vi "temp.vi"() -> ()   [LabVIEW 2018]
uses:
  <vilib>/Analysis/Matrix/Datatypes/RealMatrix.ctl
  <vilib>/myRIO/Common/Instrument Driver Framework/myRIO v1.0/PWM/vis/myRIO v1.1 Open PWM.vi
  <vilib>/myRIO/Common/Instrument Driver Framework/myRIO v1.0/PWM/vis/myRIO v1.2 Open PWM.vi
  <vilib>/myRIO/Common/Instrument Driver Framework/roboRIO v1.0/PWM/vis/roboRIO v1.0 Open PWM.vi
  <vilib>/myRIO/Common/Instrument Driver Framework/EL-RIO-CM v1.0/PWM/vis/EL-RIO-CM v1.0 Open PWM.vi
  <vilib>/myRIO/Common/Instrument Driver Framework/ELVIS III v1.0/PWM/vis/ELVIS III v1.1 Open PWM.vi
  <vilib>/myRIO/Common/Instrument Driver Framework/myRIO v1.0/UART/vis/myRIO v1.0 Close UART.vi
  <vilib>/myRIO/Common/Instrument Driver Framework/Utilities/vis/Validate Channels.vi
  <vilib>/myRIO/Common/Instrument Driver Framework/myRIO v1.0/PWM/vis/myRIO v1.0 Reserve PWM.vi
  <vilib>/myRIO/Common/Instrument Driver Framework/roboRIO v1.0/PWM/vis/roboRIO v1.0 Reserve PWM.vi
  <vilib>/myRIO/Common/Instrument Driver Framework/ELVIS III v1.0/PWM/vis/ELVIS III v1.0 Reserve PWM.vi
  <vilib>/myRIO/Common/Instrument Driver Framework/myRIO v1.0/PWM/vis/myRIO v1.0 Build MUX Configuration PWM.vi
  <vilib>/myRIO/Common/Instrument Driver Framework/myRIO v1.0/Resource Manager/vis/myRIO v1.0 Reserve Channel List.vi
  <vilib>/myRIO/Common/Instrument Driver Framework/roboRIO v1.0/PWM/vis/roboRIO v1.0 Build MUX Configuration PWM.vi
  <vilib>/myRIO/Common/Instrument Driver Framework/roboRIO v1.0/Resource Manager/vis/roboRIO v1.0 Reserve Channel List.vi
  <vilib>/myRIO/Common/Instrument Driver Framework/ELVIS III v1.0/Resource Manager/vis/ELVIS III v1.0 Reserve Channel List.vi
  <vilib>/myRIO/Common/Instrument Driver Framework/ELVIS III v1.0/PWM/vis/ELVIS III v1.0 Build MUX Configuration PWM.vi
  <vilib>/myRIO/Common/Instrument Driver Framework/myRIO v1.0/Resource Manager/vis/myRIO v1.0 Create Configuration List.vi
  <vilib>/myRIO/Common/Instrument Driver Framework/myRIO v1.0/Resource Manager/vis/myRIO v1.0 Reserve Channel.vi
  <vilib>/myRIO/Common/Instrument Driver Framework/myRIO v1.0/Resource Manager/vis/myRIO v1.0 Unreserve Channel.vi
  <vilib>/myRIO/Common/Instrument Driver Framework/roboRIO v1.0/Resource Manager/vis/roboRIO v1.0 Create Configuration List.vi
  <vilib>/myRIO/Common/Instrument Driver Framework/roboRIO v1.0/Resource Manager/vis/roboRIO v1.0 Reserve Channel.vi
  <vilib>/myRIO/Common/Instrument Driver Framework/roboRIO v1.0/Resource Manager/vis/roboRIO v1.0 Unreserve Channel.vi
  <vilib>/myRIO/Common/Instrument Driver Framework/ELVIS III v1.0/Resource Manager/vis/ELVIS III v1.0 Reserve Channel.vi
  <vilib>/myRIO/Common/Instrument Driver Framework/ELVIS III v1.0/Resource Manager/vis/ELVIS III v1.0 Unreserve Channel.vi
  <vilib>/myRIO/Common/Instrument Driver Framework/ELVIS III v1.0/Resource Manager/vis/ELVIS III v1.0 Create Configuration List.vi
  <vilib>/myRIO/Common/Instrument Driver Framework/myRIO v1.0/Resource Manager/vis/myRIO v1.0 Build Mutex Name.vi
  <vilib>/myRIO/Common/Instrument Driver Framework/roboRIO v1.0/Resource Manager/vis/roboRIO v1.0 Build Mutex Name.vi
  <vilib>/myRIO/Common/Instrument Driver Framework/ELVIS III v1.0/Resource Manager/vis/ELVIS III v1.0 Build Mutex Name.vi
  <vilib>/myRIO/Common/Instrument Driver Framework/Utilities/vis/Set_Get Target Info.vi
  <vilib>/Utility/error.llb/Error Cluster From Error Code.vi
  <vilib>/Utility/VariantDataType/GetNumericInfo.vi
  <vilib>/myRIO/Common/Instrument Driver Framework/myRIO v1.0/myRIO v1.1 Open.vi
  <vilib>/myRIO/Common/Instrument Driver Framework/Utilities/vis/IO Manager.vi
  <vilib>/myRIO/Common/Instrument Driver Framework/Utilities/vis/Configuration Manager.vi
  <vilib>/myRIO/Common/Instrument Driver Framework/myRIO v1.0/Resource Manager/vis/myRIO v1.0 Configure IO.vi
  <vilib>/myRIO/Common/Instrument Driver Framework/myRIO v1.0/myRIO v1.0 Close.vi
  <vilib>/myRIO/Common/Instrument Driver Framework/myRIO v1.0/myRIO v1.2 Open.vi
  <vilib>/myRIO/Common/Instrument Driver Framework/roboRIO v1.0/roboRIO v1.0 Open.vi
  <vilib>/myRIO/Common/Instrument Driver Framework/roboRIO v1.0/Resource Manager/vis/roboRIO v1.0 Configure IO.vi
  <vilib>/myRIO/Common/Instrument Driver Framework/EL-RIO-CM v1.0/EL-RIO-CM v1.0 Open.vi
  <vilib>/myRIO/Common/Instrument Driver Framework/ELVIS III v1.0/ELVIS III v1.1 Open.vi
  <vilib>/myRIO/Common/Instrument Driver Framework/ELVIS III v1.0/Resource Manager/vis/ELVIS III v1.0 Configure IO.vi
  <vilib>/myRIO/Common/Instrument Driver Framework/myRIO v1.0/PWM/vis/myRIO v1.0 Write PWM.vi
  <vilib>/myRIO/Common/Instrument Driver Framework/roboRIO v1.0/PWM/vis/roboRIO v1.0 Write PWM.vi
  <vilib>/myRIO/Common/Instrument Driver Framework/ELVIS III v1.0/PWM/vis/ELVIS III v1.0 Write PWM.vi
  <vilib>/myRIO/Common/Instrument Driver Framework/Utilities/vis/FPGA Ref Manager.vi
  <vilib>/myRIO/Common/Instrument Driver Framework/myRIO v1.0/IRQ/vis/myRIO v1.0 IRQ Info FGV.vi
  <vilib>/myRIO/Common/Instrument Driver Framework/myRIO v1.0/IRQ/vis/myRIO v1.0 Timer IRQ Info FGV.vi
  <vilib>/myRIO/Instrument Drivers/Utilities/Utilities.lvlib
  <vilib>/myRIO/Instrument Drivers/Onboard IO/PWM/PWM.lvlib
  <vilib>/Analysis/Matrix/NI_Matrix.lvlib
panel:
  out "offset [%FS] 2":dbl
  in  "null offset 2":bool
  out "duty cycle [%] 2":dbl
  out "pulse width [ms] 2":dbl=1.5
  in  "freq [Hz] 2":dbl=50.0
  in  "[ESC] 2":bool
  out "offset [%FS]":dbl
  in  "null offset":bool
  out "duty cycle [%]":dbl
  out "pulse width [ms]":dbl=1.5
  in  "freq [Hz]":dbl=50.0
  in  "[ESC]":bool
  in  "PWM channel 2":tag="B/PWM0"
  in  "PWM channel":tag="B/PWM0"
  out "arm picture":refnum<vi>(3d-picture)
  out "A x B 3":T1=[[1.0, 0.0, 0.0, 0.0], [0.0, 6.123233995736766e-17, 1.0, 0.0], [0.0, -1.0, 6.123233995736766e-17, 0.0], [0.0, 0.0, 0.0, 1.0]] format="%#_2g"
  out "drawing":refnum<vi>(3d-picture)
  out "x arrya":dbl[][](array[numeric])
  out "phi array":dbl[][](array[numeric])
  out "third array":dbl[][](array[numeric])
  out "second array":dbl[][](array[numeric])
  out "first":dbl[][](array[numeric])
  in  "Enter initials":string
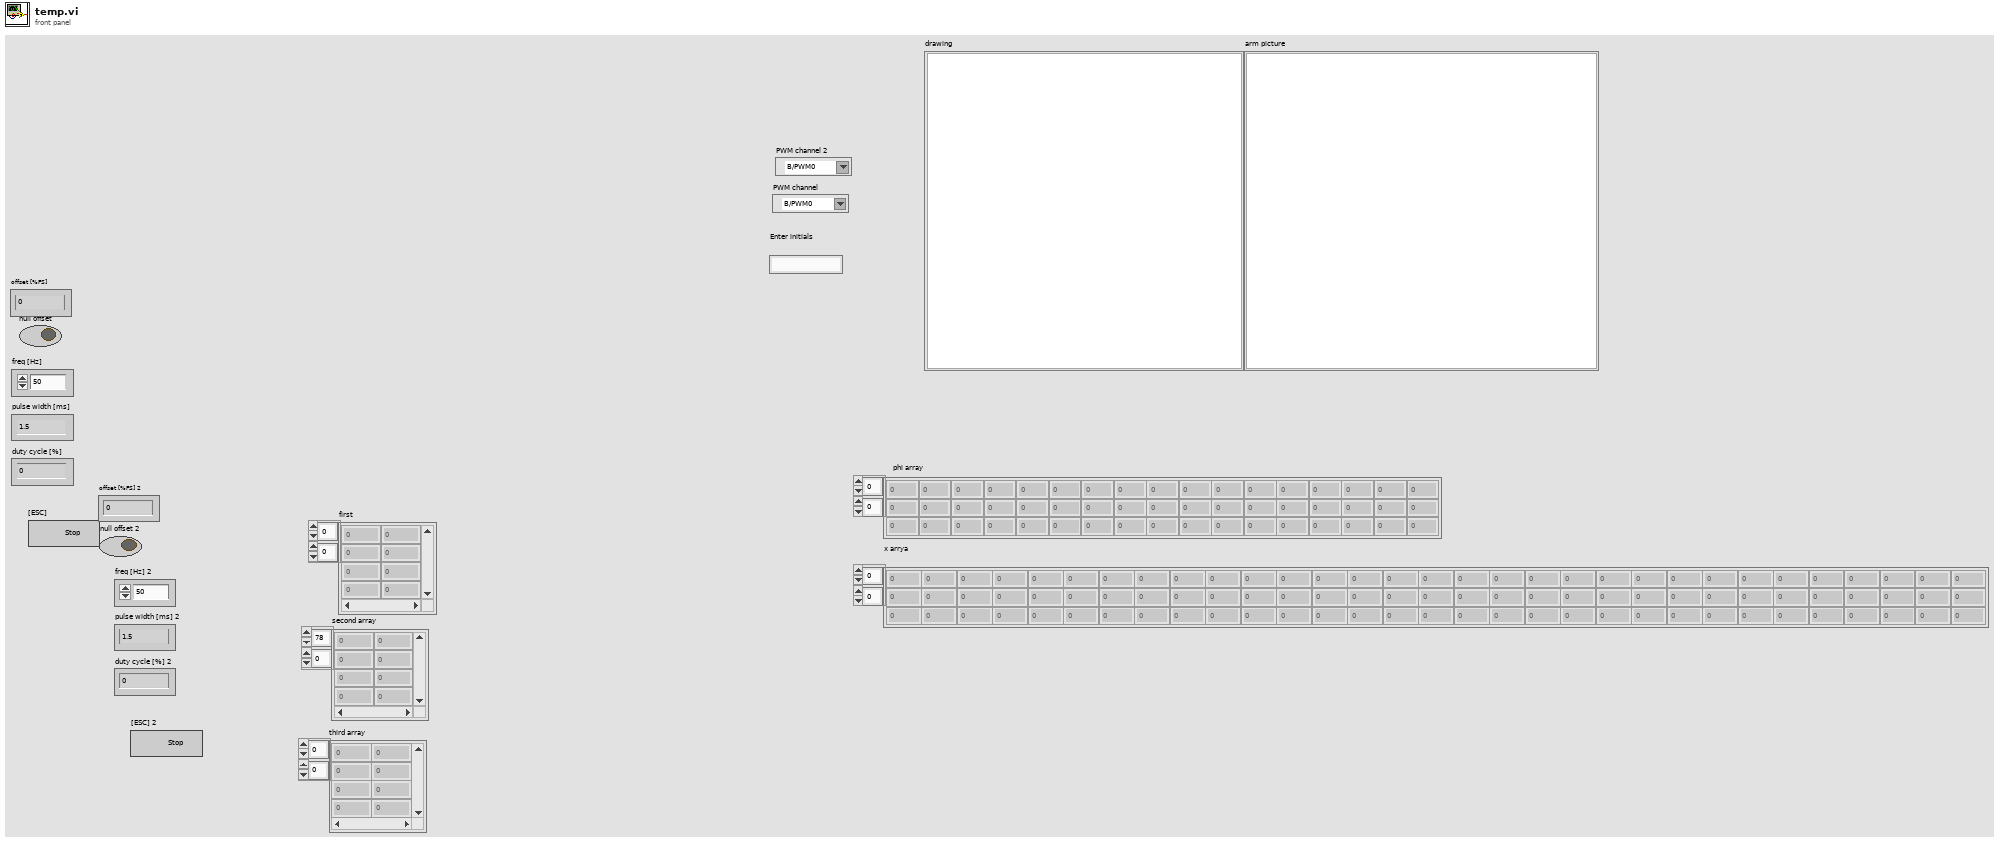
[diagram p1: front panel]
types:
  T1 = typedef "NI_Matrix.lvlib/RealMatrix.ctl" = dbl[][]
  T2 = cluster{"Theta":dbl, "d":dbl, "a":dbl, "alpha (degrees)":dbl}[]
  T3 = cluster{"Theta":dbl, "d":dbl, "a":dbl, "alpha (degrees)":dbl}
  T4 = typedef "PWM.lvlib/PWM Reference.ctl" = cluster{"myRIO Reference":T5, "PWM Channels Enum":T9, "PWM Configuration":T10}
  T5 = typedef "myRIO Generic Hardware Reference.ctl" = cluster{"myRIO Model":T6, "myRIO Hardware Reference":T7}
  T6 = typedef "Hardware Version Enum.ctl" = enum16{"Unknown", "myRIO-1900", "myRIO-1950", "roboRIO", "NI ELVIS RIO CM", "ELVIS III"}
  T7 = typedef "myRIO v1.0 Reference.ctl" = cluster{"Generic FPGA Reference":T8, "Allow multiple opens":bool}
  T8 = typedef "Generic FPGA Reference.ctl" = refnum<k20>
  T9 = typedef "PWM Channels Enum.ctl" = enum16{"Not Connected", "C/PWM0", "C/PWM1", "A/PWM0", "A/PWM1", "A/PWM2", "A/PWM3", "A/PWM4", "A/PWM5", "A/PWM6", "A/PWM7", "A/PWM8", "A/PWM9", "A/PWM10", "A/PWM11", "A/PWM12", "A/PWM13", "A/PWM14", "A/PWM15", "A/PWM16", "A/PWM17", "A/PWM18", "A/PWM19", "B/PWM0", "B/PWM1", "B/PWM2", "B/PWM3", "B/PWM4", "B/PWM5", "B/PWM6", "B/PWM7", "B/PWM8", "B/PWM9", "B/PWM10", "B/PWM11", "B/PWM12", "B/PWM13", "B/PWM14", "B/PWM15", "B/PWM16", "B/PWM17", "B/PWM18", "B/PWM19", "PWM/PWM0", "PWM/PWM1", "PWM/PWM2", "PWM/PWM3", "PWM/PWM4", "PWM/PWM5", "PWM/PWM6", "PWM/PWM7", "PWM/PWM8", "PWM/PWM9"}
  T10 = typedef "PWM.lvlib/PWM Configuration.ctl" = cluster{"Frequency":dbl, "Duty Cycle":dbl}
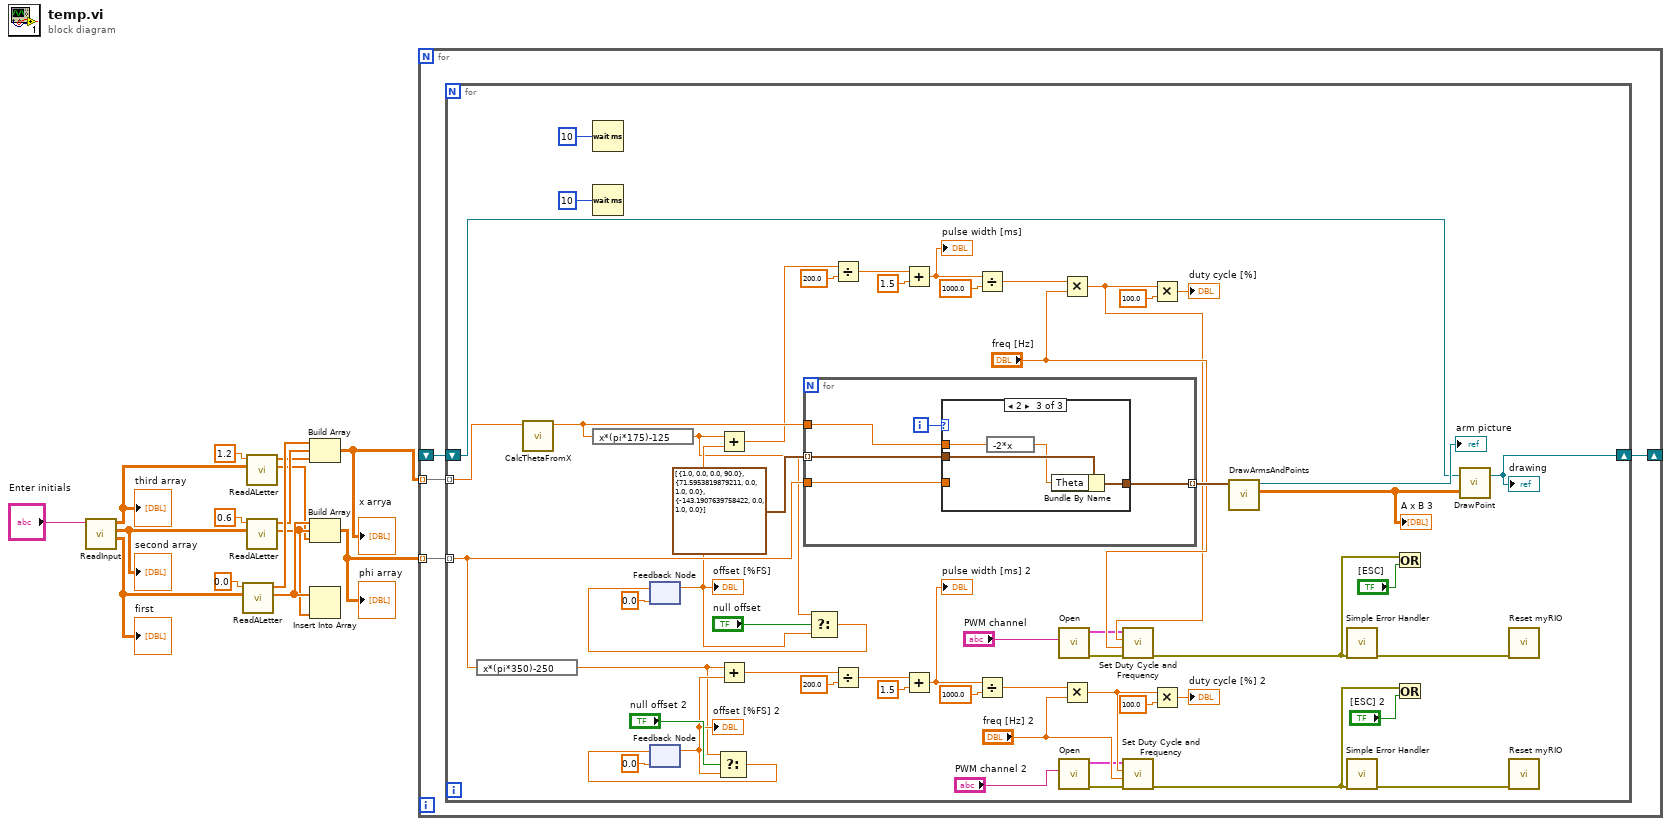
[diagram p0: block diagram]
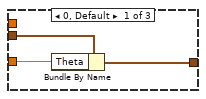
[diagram p2: hidden frame]
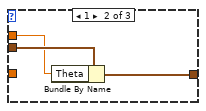
[diagram p3: hidden frame]
diagram:
  n1 = call "ReadInput.vi"("Enter initials"="Enter initials") -> ("all rows 3"=w13:dbl[][], "all rows 2"=w11:dbl[][], "all rows"=w9:dbl[][])  [unwired: 8 in]
  "first" <- w13
  "second array" <- w11
  "third array" <- w9
  n2 = call "ReadALetter.vi"("all rows 3"=w13, "x"=0.0) -> ("Array 3"=w3:dbl[], "Array 4"=w8:dbl[])  [unwired: 8 in]
  n3 = call "ReadALetter.vi"("all rows 3"=w9, "x"=1.2) -> ("Array 3"=w1:dbl[], "Array 4"=w6:dbl[])  [unwired: 8 in]
  n4 = call "ReadALetter.vi"("all rows 3"=w11, "x"=0.6) -> ("Array 3"=w2:dbl[], "Array 4"=w7:dbl[])  [unwired: 8 in]
  n5 = Build Array(w8, w7, w6) -> (w4:dbl[][])
  "x arrya" <- w4
  n6 = Build Array(w3, w2, w1) -> (w5:dbl[][])
  "phi array" <- w5
  n7 = Insert Into Array(array=w3, new element=w2) -> ()  [unwired: 1 in, 1 out]
  n8 = for {
    tunnel: w5 -> [w18] mode=indexing
    shift-right: [w19] -> _
    shift-left: _ -> [w16]
    tunnel: w4 -> [w17] mode=indexing
    n9 = for {
      tunnel: w18 -> [w62] mode=indexing
      tunnel: w17 -> [w69] mode=indexing
      shift-right: [w71] -> w19
      shift-left: w16 -> [w68]
      n10 = expression code="x*(pi*350)-250"(w62) -> (w23:dbl)
      n11 = call "CalcThetaFromX.vi"("X"=w69) -> ("Numeric"=w63:dbl)  [unwired: 10 in]
      n12 = Wait (ms)(milliseconds to wait=u32 10) -> ()  [unwired: 1 out]
      n13 = Wait (ms)(milliseconds to wait=u32 10) -> ()  [unwired: 1 out]
      n14 = expression code="x*(pi*175)-125"(w63) -> (w44:dbl)
      n15 = feedback #1(0.0 ("position [%FS]")) -> (w50:dbl)
      "offset [%FS]" <- w50
      n16 = feedback #2(0.0 ("position [%FS]")) -> (w29:dbl)
      "offset [%FS] 2" <- w29
      n17 = Select(t=w23, s="null offset 2", f=w29) -> (s? t:f=w31:dbl)
      n18 = feedback-in #2(w31) -> ()
      n19 = Add(x=w44, y=w50) -> (x+y=w51:dbl)
      n20 = Add(x=w23, y=w29) -> (x+y=w30:dbl)
      n21 = for {
        tunnel: T2 [{"Theta"=1.0, "d"=0.0, "a"=0.0, "alpha (degrees)"=90.0}, {"Theta"=71.5953819879211, "d"=0.0, "a"=1.0, "alpha (degrees)"=0.0}, {"Theta"=-143.1907639758422, "d"=0.0, "a"=1.0, "alpha (degrees)"=0.0}] ("Joints") -> [w79] mode=indexing
        tunnel: [w78] -> w73 mode=indexing
        tunnel: w63 -> [w76]
        tunnel: w62 -> [w75]
        i -> [w77]
        n22 = case shown="2" w77 {
          tunnel: w76 -> [_ w84 w88]
          tunnel: w79 -> [w82 w85 w89]
          tunnel: [w80 w83 w87] -> w78
          tunnel: w75 -> [w81 _ _]
          frame 0, Default {
            n23 = Bundle By Name(cluster=w82, "Theta"=w81) -> (w80:T3)
          }
          frame 1 {
            n24 = Bundle By Name(cluster=w85, "Theta"=w84) -> (w83:T3)
          }
          frame 2 {
            n25 = expression code="-2*x"(w88) -> (w86:dbl)
            n26 = Bundle By Name(cluster=w89, "Theta"=w86) -> (w87:T3)
          }
        }
      }
      n27 = Select(t=w44, s="null offset", f=w50) -> (s? t:f=w52:dbl)
      n28 = feedback-in #1(w52) -> ()
      n29 = Divide(x=w51, y=200.0) -> (x/y=w58:dbl)
      n30 = Divide(x=w30, y=200.0) -> (x/y=w37:dbl)
      n31 = Add(x=w58, y=1.5) -> (x+y=w56:dbl)
      "pulse width [ms]" <- w56
      n32 = Add(x=w37, y=1.5) -> (x+y=w35:dbl)
      "pulse width [ms] 2" <- w35
      n33 = Divide(x=w56, y=1000.0) -> (x/y=w49:dbl)
      n34 = Divide(x=w35, y=1000.0) -> (x/y=w28:dbl)
      n35 = call <vilib>:"Open.vi"("Channel Name"="PWM channel") -> ("error out"=w42:errorcluster, "PWM Ref Out"=w43:T4)  [unwired: 9 in]
      n36 = call <vilib>:"Open.vi"("Channel Name"="PWM channel 2") -> ("error out"=w21:errorcluster, "PWM Ref Out"=w22:T4)  [unwired: 9 in]
      n37 = Multiply(x=w49, y="freq [Hz]") -> (x*y=w46:dbl)
      n38 = Multiply(x=w28, y="freq [Hz] 2") -> (x*y=w25:dbl)
      n39 = call <vilib>:"Set Duty Cycle and Frequency.vi"("error in (no error)"=w42, "Frequency [Hz]"="freq [Hz]", "Duty Cycle"=w46, "PWM Ref In"=w43) -> ("error out"=w41:errorcluster)  [unwired: 5 in, 1 out]
      n40 = call <vilib>:"Set Duty Cycle and Frequency.vi"("error in (no error)"=w21, "Frequency [Hz]"="freq [Hz] 2", "Duty Cycle"=w25, "PWM Ref In"=w22) -> ("error out"=w20:errorcluster)  [unwired: 5 in, 1 out]
      n41 = Multiply(x=w46, y=100.0) -> (x*y=→"duty cycle [%]":dbl)
      n42 = Multiply(x=w25, y=100.0) -> (x*y=→"duty cycle [%] 2":dbl)
      n43 = call "DrawArmsAndPoints.vi"("Array"=w73) -> ("A x B"=w72:T1, "SceneObject out"=→"arm picture":refnum<vi>)  [unwired: 9 in]
      "A x B 3" <- w72
      n44 = call <vilib>:"Simple Error Handler.vi"("error in (no error)"=w41) -> ("error out"=w67:errorcluster)  [unwired: 4 in, 4 out]
      n45 = call <vilib>:"Simple Error Handler.vi"("error in (no error)"=w20) -> ("error out"=w65:errorcluster)  [unwired: 4 in, 4 out]
      n46 = Or(x=w41, y="[ESC]") -> ()  [unwired: 1 out]
      n47 = Or(x=w20, y="[ESC] 2") -> ()  [unwired: 1 out]
      n48 = call "DrawPoint.vi"("Start"=w72, "Stage in"=w68) -> ("Stage out"=w71:refnum<vi>)  [unwired: 1 in]
      "drawing" <- w71
      n49 = call <vilib>:"Reset myRIO.vi"("error in (no error)"=w67) -> ()  [unwired: 10 in, 1 out]
      n50 = call <vilib>:"Reset myRIO.vi"("error in (no error)"=w65) -> ()  [unwired: 10 in, 1 out]
    }
  }
